vi "Acquire.vi"(6 "Acquisition":refnum<queue>, 7 "Longueur d'onde":dbl, 8 "error in (no error)":errorcluster, 9 "Data Queue":refnum<queue>, 10 "Data Notifier":refnum<notifier>, 11 "Loop Count":dbl) -> (0 "error out":errorcluster, 3 "Disconnected":bool=TRUE)   [LabVIEW 2018, in "Acquisition.lvlib"]
doc: "Perform the acquisition. Replace the contents of this diagram with calls to acquisition hardware."
uses:
  Acquisition.lvlib
  support/Message Queue/Message Cluster.ctl
  support/Message Queue/Message Queue.lvlib
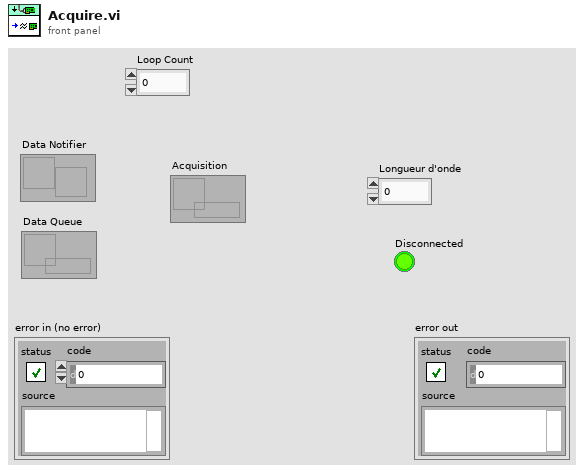
[diagram p1: front panel]
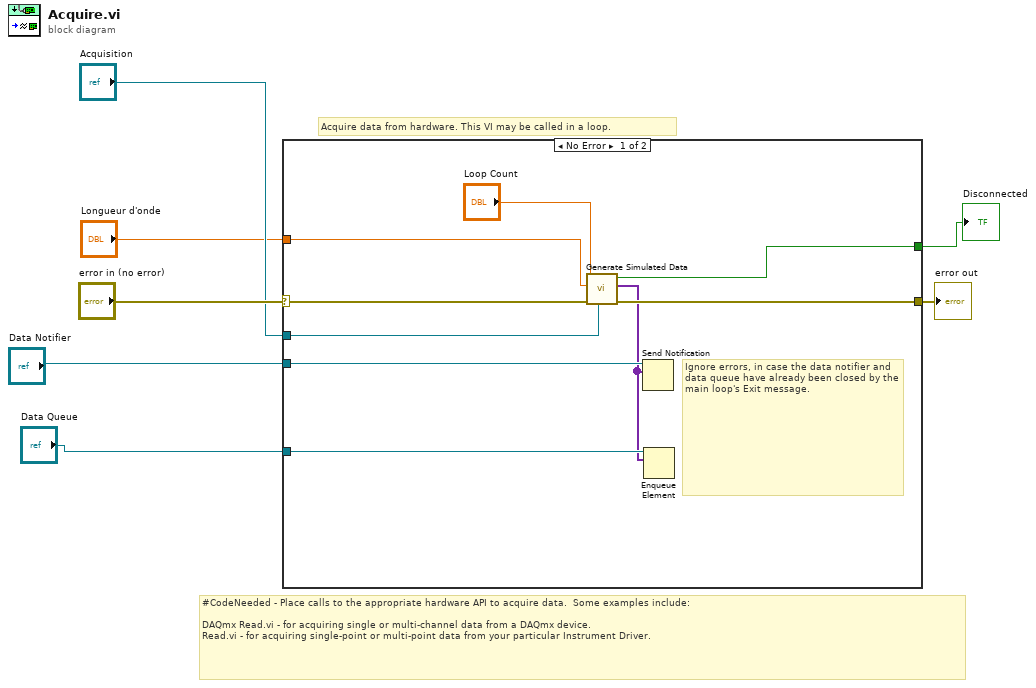
[diagram p0: block diagram]
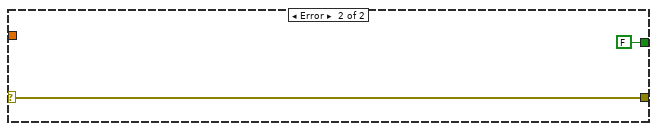
[diagram p2: hidden frame]
diagram:
  # "Acquire data from hardware. This VI may be called in a loop."
  # "#CodeNeeded - Place calls to the appropriate hardware API to acquire data.  Some examples include:\n\nDAQmx Read.vi - for acquiring single or multi-channel data from a DAQmx device.\nRead.vi - for acquiring single-point or multi-point data from your particular Instrument Driver."
  n1 = case shown="No Error" "error in (no error)" {
    selector: "error in (no error)" -> [w16 w18]
    tunnel: [w13 w18] -> w6
    tunnel: "Data Notifier" -> [w15 _]
    tunnel: "Data Queue" -> [w14 _]
    tunnel: "Acquisition" -> [w12 _]
    tunnel: "Longueur d'onde" -> [w11 _]
    tunnel: [w9 FALSE ("Disconnected")] -> w1
    frame No Error {
      # "Ignore errors, in case the data notifier and data queue have already been closed by the main loop's Exit message."
      n2 = call "Generate Simulated Data.vi"("Acquisition"=w12, "error in (no error)"=w16, "Longueur d'onde"=w11, "Loop Count"="Loop Count") -> ("error out"=w13:errorcluster, "Data Out"=w10:variant[], "Disconnected"=w9:bool)  [unwired: 5 in]
      n3 = Send Notification(notification=w10, notifier=w15) -> ()  [unwired: 1 in, 2 out]
      n4 = Enqueue Element(queue=w14, element=w10) -> ()  [unwired: 2 in, 3 out]
    }
    frame Error {
    }
  }
  "error out" <- w6
  "Disconnected" <- w1
